vi "客户端侦听列表.vi"() -> ()   [LabVIEW 2016, in "wxpusher.lvlib"]
uses:
  wxpusher.lvlib
  <vilib>/Utility/miscctls.llb/LVPointTypeDef.ctl
  <vilib>/regexp/Match Regular Expression.xnode
panel:
  in  "开机启动":bool
  out "remote port":u16
  out "remote address":string
  out "data out":string
  out "数组":refnum<k5>[](array[refnum])
  out "回调信息":T1
  out "侦听列表":T2(array[cluster])
  in  "客户端列表":i32(listbox)
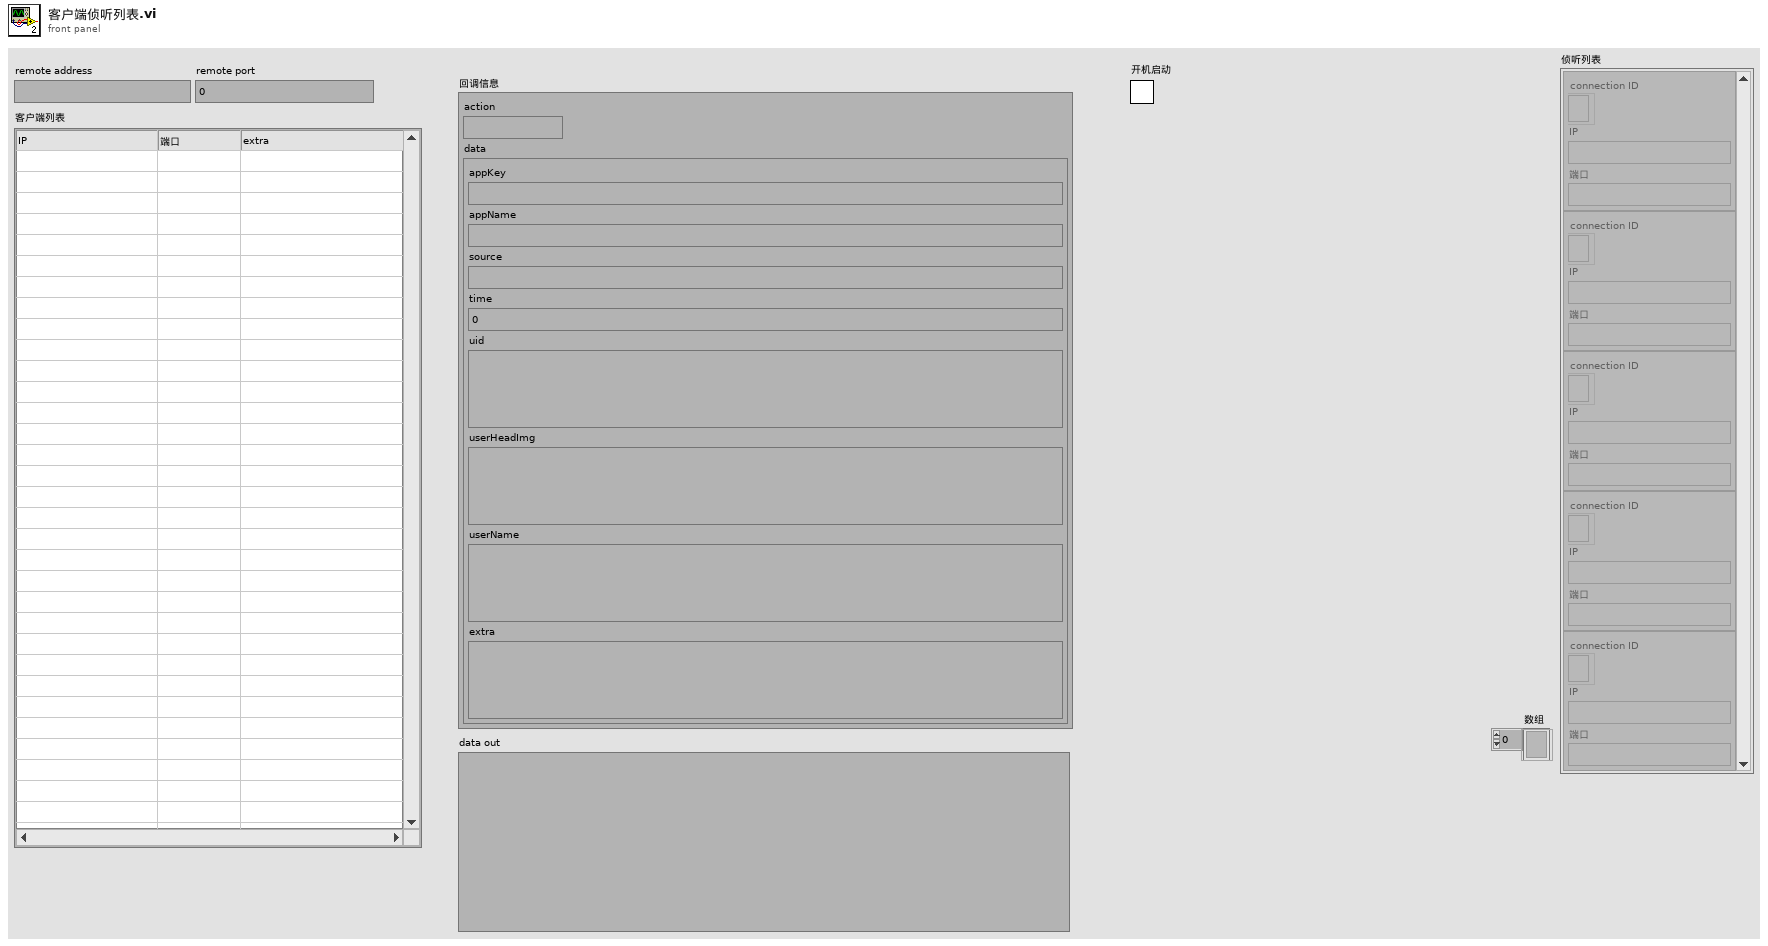
[diagram p1: front panel]
types:
  T1 = cluster{"action":string, "data":cluster{"appKey":string, "appName":string, "source":string, "time":u64, "uid":string, "userHeadImg":string, "userName":string, "extra":string}}
  T2 = cluster{"connection ID":refnum<k5>, "IP":string, "端口":string}[]
  T3 = typedef "LVPointTypeDef.ctl" = cluster{"Horizontal":i16, "Vertical":i16}
  T4 = cluster{"数据输出":string, "data":cluster{"action":string, "data":cluster{"appKey":string, "appName":string, "source":string, "time":u64, "uid":string, "userHeadImg":string, "userName":string, "extra":string}}}
  T5 = cluster{"connection ID":refnum<k5>, "IP":string, "端口":string}
  T6 = enum16{"Standard", "Buffered", "CRLF", "Immediate"}
  T7 = cluster{"data out":string, "类型和默认值":cluster{"action":string, "data":cluster{"appKey":string, "appName":string, "source":string, "time":u64, "uid":string, "userHeadImg":string, "userName":string, "extra":string}}}
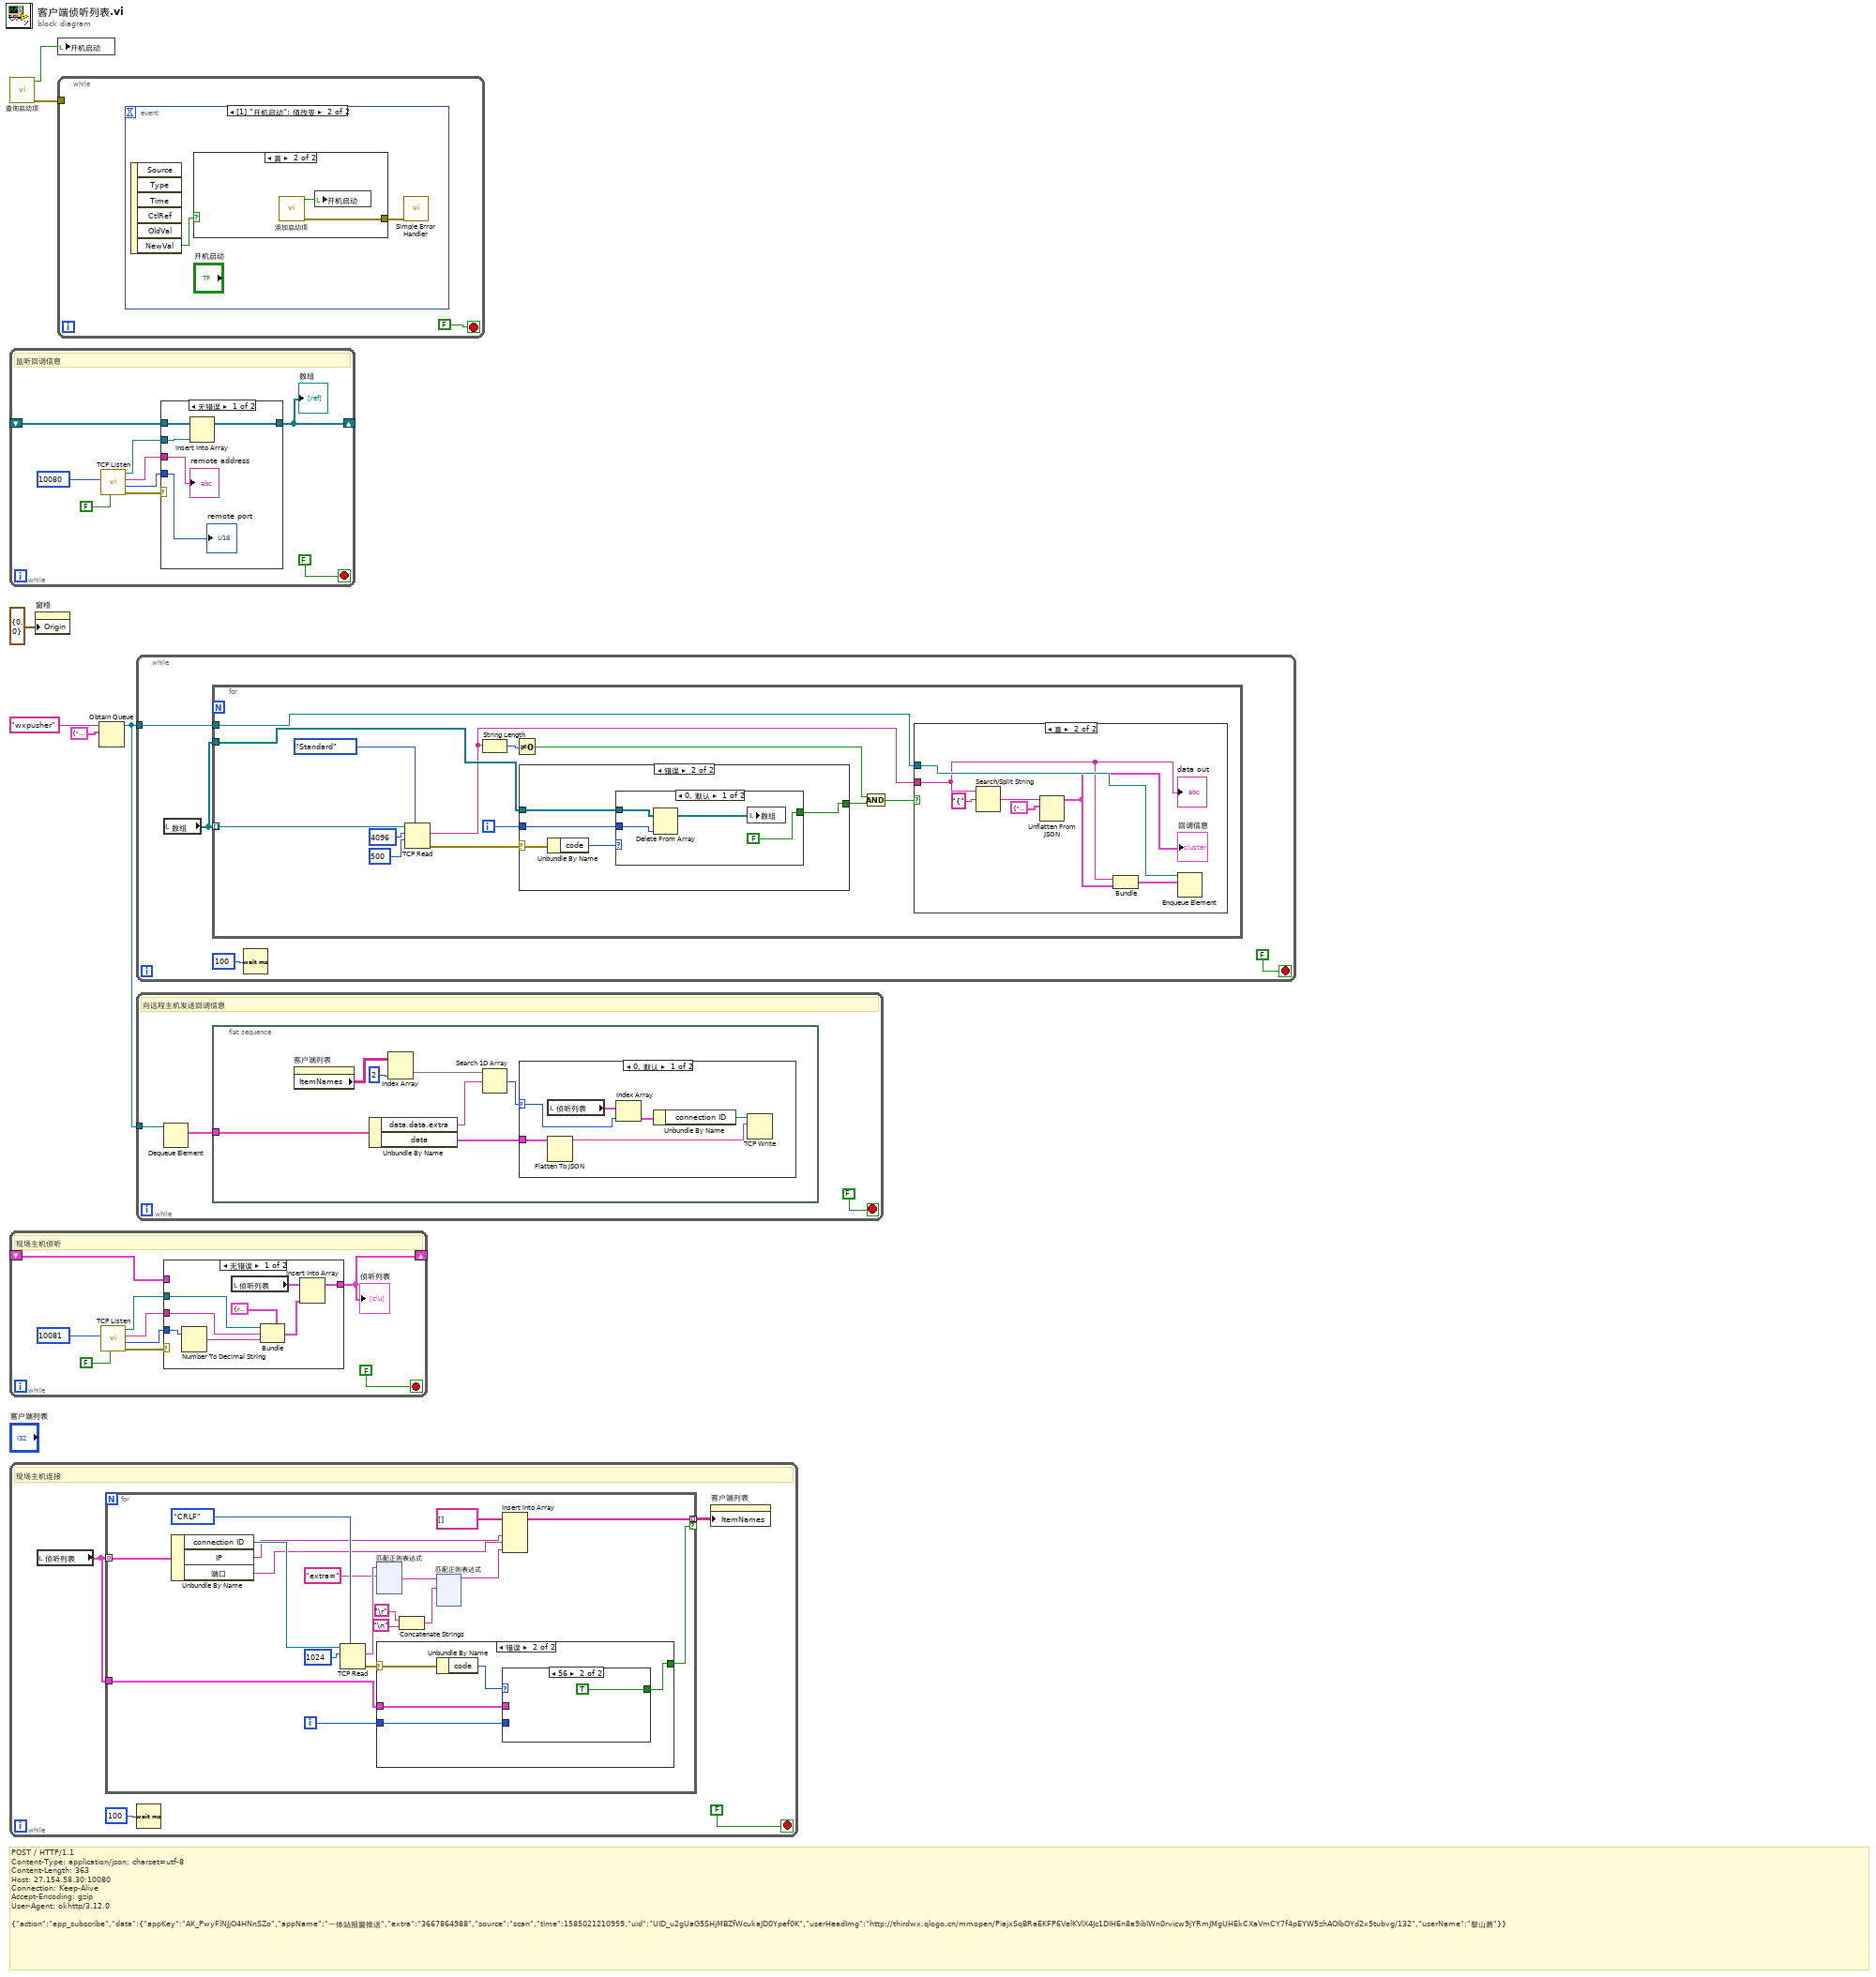
[diagram p0: block diagram]
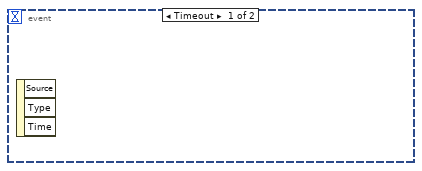
[diagram p2: hidden frame]
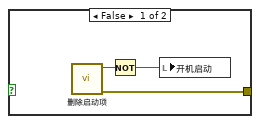
[diagram p3: hidden frame]
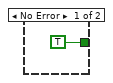
[diagram p5: hidden frame]
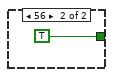
[diagram p6: hidden frame]
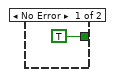
[diagram p9: hidden frame]
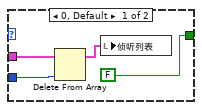
[diagram p10: hidden frame]
diagram:
  # "POST / HTTP/1.1\nContent-Type: application/json; charset=utf-8\nContent-Length: 363\nHost: 27.154.58.30:10080\nConnection: Keep-Alive\nAccept-Encoding: gzip\nUser-Agent: okhttp/3.12.0\n\n{\"action\":\"app_subscribe\",\"data\":{\"appKey\":\"AK_PwyFlNJjO4HNnSZo\",\"appName\":\"一体站报警推送\",\"extra\":\"3667864988\",\"source\":\"scan\",\"time\":1585021210959,\"uid\":\"UID_u2gUaG5SHjMBZfWcukaJD0Ypef0K\",\"userHeadImg\":\"http://thirdwx.qlogo.cn/mmopen/PiajxSqBRaEKFP6VelKVlX4Jc1DIHEn8a9ibIWn0rvicw9jYRmJMgUHEkCXaVmCY7f4pEYW5zhAOIbOYd2x5tubvg/132\",\"userName\":\"黎山萧\"}}"
  n1 = call "查询启动项.vi"() -> ("error out"=w3:errorcluster, "包含启动项"=w2:bool)  [unwired: 9 in, 1 out]
  n2 = while {
    shift-right: [w10] -> _
    shift-left: _ -> [w9]
    stop <- FALSE stop-if-true
    # "监听回调信息"
    n3 = call <vilib>:"TCP Listen.vi"("resolve remote address (T)"=FALSE, "port"=u16 10080) -> ("error out"=w13:errorcluster, "remote port"=w7:u16, "remote address"=w12:string, "connection ID"=w11:refnum<k5>)  [unwired: 5 in, 1 out]
    n4 = case shown="无错误" w13 {
      tunnel: w11 -> [w20 _]
      tunnel: w12 -> [w17 _]
      tunnel: [w19 w21] -> w10
      tunnel: w9 -> [w18 w21]
      tunnel: w7 -> [w16 _]
      frame No Error {
        n5 = Insert Into Array(array=w18, new element=w20) -> (w19:refnum<k5>[])  [unwired: 1 in]
        "remote address" <- w17
        "remote port" <- w16
      }
      frame Error {
      }
    }
    "数组" <- w10
  }
  n6 = while {
    shift-right: [w24] -> _
    shift-left: _ -> [w23]
    stop <- FALSE stop-if-true
    # "现场主机侦听"
    n7 = call <vilib>:"TCP Listen.vi"("resolve remote address (T)"=FALSE, "port"=u16 10081) -> ("error out"=w28:errorcluster, "remote port"=w25:u16, "remote address"=w26:string, "connection ID"=w27:refnum<k5>)  [unwired: 5 in, 1 out]
    n8 = case shown="无错误" w28 {
      tunnel: w27 -> [w38 _]
      tunnel: w26 -> [w32 _]
      tunnel: w25 -> [w33 _]
      tunnel: [w36 w39] -> w24
      tunnel: w23 -> [_ w39]
      frame No Error {
        n9 = Number To Decimal String(number=w33) -> (decimal integer string=w35:string)  [unwired: 1 in]
        n10 = local read "侦听列表"() -> (w31:T2)
        n11 = Bundle(cluster=T5 {"connection ID"=refnum, "IP"="", "端口"=""} ("簇"), "connection ID"=w38, "IP"=w32, "端口"=w35) -> (w37:T5)
        n12 = Insert Into Array(array=w31, new element=w37) -> (w36:T2)  [unwired: 1 in]
      }
      frame Error {
      }
    }
    "侦听列表" <- w24
  }
  n13 = while {
    stop <- FALSE stop-if-true
    # "现场主机连接"
    n14 = local read "侦听列表"() -> (w41:T2)
    n15 = for {
      tunnel: w41 -> [w62] mode=indexing
      tunnel: [w44] -> w40 mode=indexing if=w49
      tunnel: w41 -> [w51]
      i -> [w50]
      n16 = Unbundle By Name(w62) -> ("connection ID"=w61:refnum<k5>, "IP"=w48:string, "端口"=w47:string)
      n17 = TCP Read(connection ID=w61, bytes to read=1024 ("读取的字节"), 7:T6."CRLF" ("模式（标准）")) -> (data out=w58:string, error out=w52:errorcluster)  [unwired: 2 in, 1 out]
      n18 = xnode "匹配正则表达式"("输入字符串"=w58, "正则表达式"="extra=") -> ("匹配之后"=w56:string)  [unwired: 4 in, 4 out]
      n19 = case shown="错误" w52 {
        selector: w52 -> [_ w68]
        tunnel: w51 -> [_ w66]
        tunnel: w50 -> [_ w65]
        tunnel: [TRUE w64] -> w49
        frame No Error {
        }
        frame Error {
          n20 = Unbundle By Name(w68) -> ("code"=w67:i32)
          n21 = case shown="56" w67 {
            tunnel: w66 -> [w72 _]
            tunnel: w65 -> [w71 _]
            tunnel: [FALSE TRUE] -> w64
            frame 0, Default {
              n22 = Delete From Array(array=w72, index=w71) -> (array with subset deleted=w70:T2)  [unwired: 1 in, 1 out]
              n23 = local write "侦听列表"(w70) -> ()
            }
            frame 56 {
            }
          }
        }
      }
      n24 = Concatenate Strings("\r", "\n") -> (w53:string)
      n25 = xnode "匹配正则表达式"("输入字符串"=w56, "正则表达式"=w53) -> ("匹配之前"=w46:string)  [unwired: 4 in, 4 out]
      n26 = Insert Into Array(array=string[] [] ("数组"), new element #1=w48, new element #2=w47, new element #3=w46) -> (w44:string[])  [unwired: 1 in]
    }
    n27 = Wait (ms)(milliseconds to wait=u32 100 ("等待时间（毫秒）")) -> ()  [unwired: 1 out]
    n28 = property on="客户端列表" class="MCListbox (严格)"("ItemNames"=w40) -> ()  [unwired: 2 in, 2 out]
  }
  n29 = property on="窗格" class="Pane"("Origin"=T3 {"Horizontal"=0, "Vertical"=0} ("原点")) -> ()  [unwired: 2 in, 2 out]
  n30 = local write "开机启动"(w2) -> ()
  n31 = while {
    tunnel: w3 -> [_]
    stop <- FALSE stop-if-true
    n32 = event shown="[1] \"开机启动\": 值改变" {
      selector: _ -> [_ _]
      dyn-events: _ -> [_ _]
      timeout: _ -> [_ _]
      event Timeout {
        n33 = event-data() -> ()  [unwired: 1 in, 3 out]
      }
      event "开机启动": Value Change {
        n34 = event-data() -> ("NewVal"=w304:bool)  [unwired: 1 in, 5 out]
        n35 = case shown="真" w304 {
          tunnel: [w305 w308] -> w303
          frame False {
            n36 = call "删除启动项.vi"() -> ("error out"=w305:errorcluster, "删除标记"=w307:bool)  [unwired: 10 in]
            n37 = Not(x=w307) -> (.not. x?=w306:bool)
            n38 = local write "开机启动"(w306) -> ()
          }
          frame True {
            n39 = call "添加启动项.vi"() -> ("error out"=w308:errorcluster, "添加成功标记"=w309:bool)  [unwired: 10 in]
            n40 = local write "开机启动"(w309) -> ()
          }
        }
        n41 = call <vilib>:"Simple Error Handler.vi"("error in (no error)"=w303) -> ()  [unwired: 4 in, 5 out]
      }
    }
  }
  n42 = Obtain Queue(name (unnamed)="wxpusher" ("名称（未命名）"), element data type=T4 {"数据输出"="", "data"={"action"="", "data"={"appKey"="", "appName"="", "source"="", "time"=0, "uid"="", "userHeadImg"="", "userName"="", "extra"=""}}}) -> (queue out=w4:refnum<queue>)  [unwired: 3 in, 2 out]
  n43 = while {
    tunnel: w4 -> [w312]
    stop <- FALSE stop-if-true
    n44 = local read "数组"() -> (w310:refnum<k5>[])
    n45 = for {
      tunnel: w312 -> [w326]
      tunnel: w310 -> [w322] mode=indexing
      tunnel: w310 -> [w319]
      i -> [w321]
      n46 = TCP Read(connection ID=w322, bytes to read=4096 ("读取的字节"), 7:T6."Standard" ("模式（标准）"), 9:500 ("超时毫秒(25000)")) -> (data out=w317:string, error out=w320:errorcluster)  [unwired: 1 in, 1 out]
      n47 = String Length(string=w317) -> (length=w316:i32)
      n48 = Not Equal To 0?(x=w316) -> (x != 0?=w314:bool)
      n49 = case shown="错误" w320 {
        selector: w320 -> [_ w339]
        tunnel: w319 -> [_ w337]
        tunnel: w321 -> [_ w336]
        tunnel: [TRUE w335] -> w318
        frame No Error {
        }
        frame Error {
          n50 = Unbundle By Name(w339) -> ("code"=w338:i32)
          n51 = case shown="0, 默认" w338 {
            tunnel: w337 -> [w343 _]
            tunnel: w336 -> [w342 _]
            tunnel: [FALSE TRUE] -> w335
            frame 0, Default {
              n52 = Delete From Array(array=w343, index=w342) -> (array with subset deleted=w341:refnum<k5>[])  [unwired: 1 in, 1 out]
              n53 = local write "数组"(w341) -> ()
            }
            frame 56 {
            }
          }
        }
      }
      n54 = And(x=w314, y=w318) -> (x .and. y?=w315:bool)
      n55 = case shown="真" w315 {
        tunnel: w326 -> [_ w333]
        tunnel: w317 -> [_ w332]
        frame False {
        }
        frame True {
          n56 = Search/Split String(string=w332, search string/char (-)="{" ("搜索字符串/字符(-)")) -> (match + rest of string=w329:string)  [unwired: 1 in, 2 out]
          n57 = Unflatten From JSON(JSON string=w329, type and defaults=T1 {"action"="", "data"={"appKey"="", "appName"="", "source"="", "time"=0, "uid"="", "userHeadImg"="", "userName"="", "extra"=""}} ("类型和默认值")) -> (value=w328:T1)  [unwired: 5 in, 1 out]
          "回调信息" <- w328
          n58 = Bundle("data out"=w332, "类型和默认值"=w328) -> (w327:T7)  [unwired: 1 in]
          n59 = Enqueue Element(queue=w333, element=w327) -> ()  [unwired: 2 in, 3 out]
          "data out" <- w332
        }
      }
    }
    n60 = Wait (ms)(milliseconds to wait=u32 100 ("等待时间（毫秒）")) -> ()  [unwired: 1 out]
  }
  n61 = while {
    tunnel: w4 -> [w347]
    stop <- FALSE stop-if-true
    # "向远程主机发送回调信息"
    n62 = Dequeue Element(queue=w347) -> (element=w345:T4)  [unwired: 2 in, 3 out]
    n63 = flat-sequence {
      tunnel: w345 -> [w354]
      frame #0 {
        n64 = property on="客户端列表" class="MCListbox (严格)"() -> ("ItemNames"=w353:string[][])  [unwired: 2 in, 2 out]
        n65 = Unbundle By Name(w354) -> ("data.data.extra"=w350:string, "data"=w348:T1)
        n66 = Index Array(array=w353, index (col)=2 ("禁用的索引 (列)")) -> (element=w351:string[])  [unwired: 1 in]
        n67 = Search 1D Array(1D array=w351, element=w350) -> (index of element=w349:i32)  [unwired: 1 in]
        n68 = case shown="0, 默认" w349 {
          selector: w349 -> [w359 _]
          tunnel: w348 -> [w358 _]
          frame 0, Default {
            n69 = local read "侦听列表"() -> (w360:T2)
            n70 = Flatten To JSON(anything=w358) -> (JSON string=w355:string)  [unwired: 2 in, 1 out]
            n71 = Index Array(array=w360, index=w359) -> (element=w357:T5)
            n72 = Unbundle By Name(w357) -> ("connection ID"=w356:refnum<k5>)
            n73 = TCP Write(connection ID=w356, data in=w355) -> ()  [unwired: 2 in, 3 out]
          }
          frame -1 {
          }
        }
      }
    }
  }
